vi "ToggleCheck.vi"(10 "button in":bool) -> (2 "toggled?":bool)   [LabVIEW 2019]
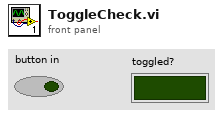
[diagram p1: front panel]
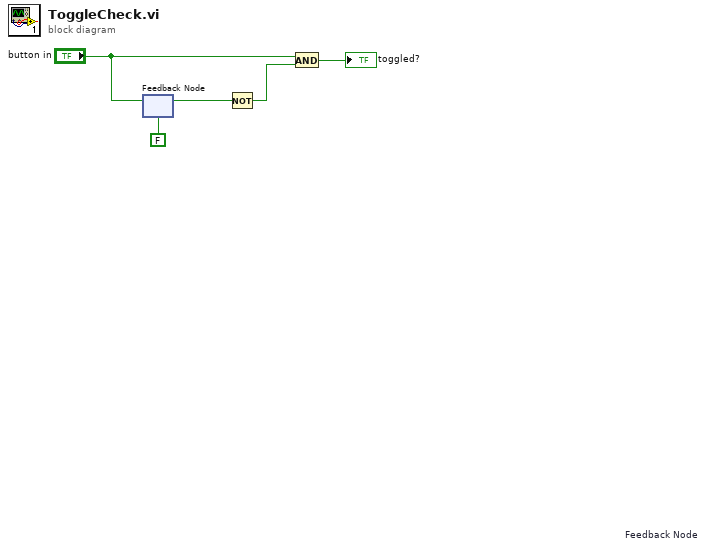
[diagram p0: block diagram]
diagram:
  n1 = feedback #1 "Feedback Node"(FALSE ("Button In")) -> (w5:bool)
  n2 = feedback-in #1("button in") -> ()
  n3 = Not(x=w5) -> (.not. x?=w4:bool)
  n4 = And(x="button in", y=w4) -> (x .and. y?=→"toggled?":bool)
